vi "get_IMAQdxSession.vi"(3 "error in (no error)":errorcluster, 5 "HGF_ImaqDx in":refnum<class "HGF_ImaqDx.lvclass">) -> (0 "error out":errorcluster, 1 "IMAQdx Session":T1, 2 "HGF_ImaqDx out":refnum<class "HGF_ImaqDx.lvclass">)   [LabVIEW 2014, in "HGF_IMAQ.lvlib" / "HGF_ImaqDx.lvclass"]
doc: "Returns member: IMAQdx Session."
uses:
  HGF_ImaqDx.lvclass
  <vilib>/userdefined/High Color/IMAQdx.ctl
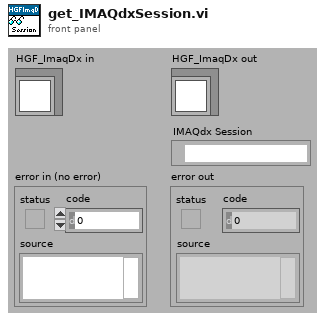
[diagram p1: front panel]
types:
  T1 = typedef "IMAQdx.ctl" = refnum<k21>
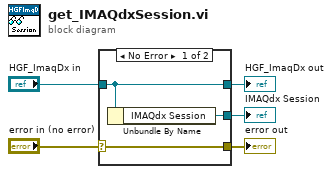
[diagram p0: block diagram]
diagram:
  n1 = case shown="No Error" "error in (no error)" {
    selector: "error in (no error)" -> [w8 w9]
    tunnel: [w8 w9] -> w4
    tunnel: [w7 w10] -> w2
    tunnel: "HGF_ImaqDx in" -> [w7 w10]
    tunnel: [w6 _] -> w1
    frame No Error {
      n2 = Unbundle By Name(w7) -> ("IMAQdx Session"=w6:T1)
    }
    frame Error {
    }
  }
  "error out" <- w4
  "HGF_ImaqDx out" <- w2
  "IMAQdx Session" <- w1
